vi "isi.vi"() -> ()   [LabVIEW 2019]
uses:
  <vilib>/DAQmx/write.llb/DAQmx Write (Digital Bool 1Line 1Point).vi
  <vilib>/DAQmx/read.llb/DAQmx Read (Analog 1D Wfm NChan NSamp).vi
  <vilib>/DAQmx/write.llb/DAQmx Write (Analog 1D DBL 1Chan NSamp).vi
  <vilib>/DAQmx/create/channels.llb/DAQmx Create Channel (DO-Digital Output).vi
  <vilib>/DAQmx/miscellaneous.llb/DAQmx Fill In Error Info.vi
  <vilib>/DAQmx/create/channels.llb/DAQmx Create Channel (AO-Voltage-Basic).vi
  <vilib>/DAQmx/configure/timing.llb/DAQmx Timing (Sample Clock).vi
  <vilib>/DAQmx/create/channels.llb/DAQmx Create Channel (AI-Voltage-Basic).vi
  <vilib>/DAQmx/configure/task.llb/DAQmx Configure Logging (TDMS).vi
  <vilib>/measure/NI_MABase.lvlib
panel:
  in  "确定按钮":bool
  in  "lines":tag="Dev2/port0/line0" caption="事件通道"
  in  "logging mode":i32(ring)=10231 caption="记录模式" items=["关"=10231, "记录"=15844, "记录并读取"=15842]
  out "波形图":waveform(dbl)[](graph)
  in  "samples per channel":i32=1000 caption="每通道采样"
  in  "physical channels":tag="Dev2/ai0:3" caption="输入通道"
  in  "file path":path caption="文件路径"
  in  "停止 2":bool
  in  "lines 2":tag="Dev2/port0/line1" caption="刺激事件通道"
  in  "胡须刺激":bool
  in  "frequency":dbl=10.0 caption="刺激频率" format="%0.2p"
  in  "amplitude":dbl=2.5 caption="刺激幅值" format="%0.2p"
  in  "physical channels 3":tag="Dev2/ao1" caption="胡须刺激通道"
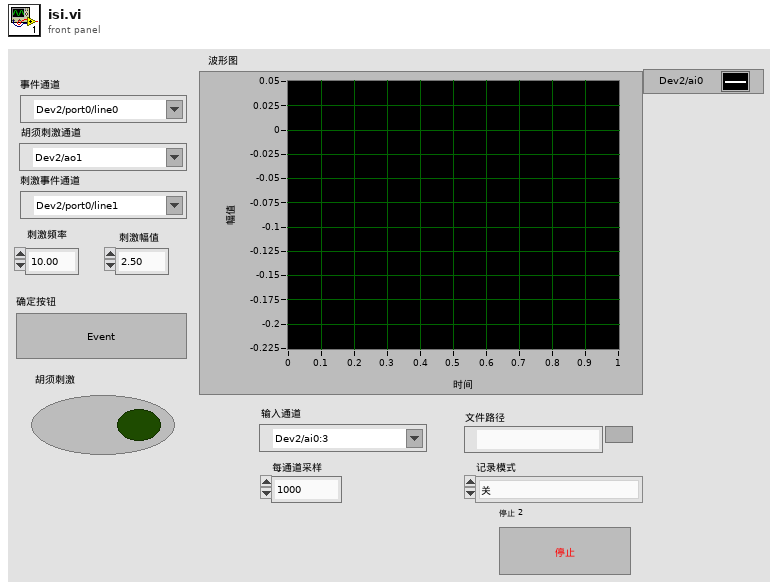
[diagram p1: front panel]
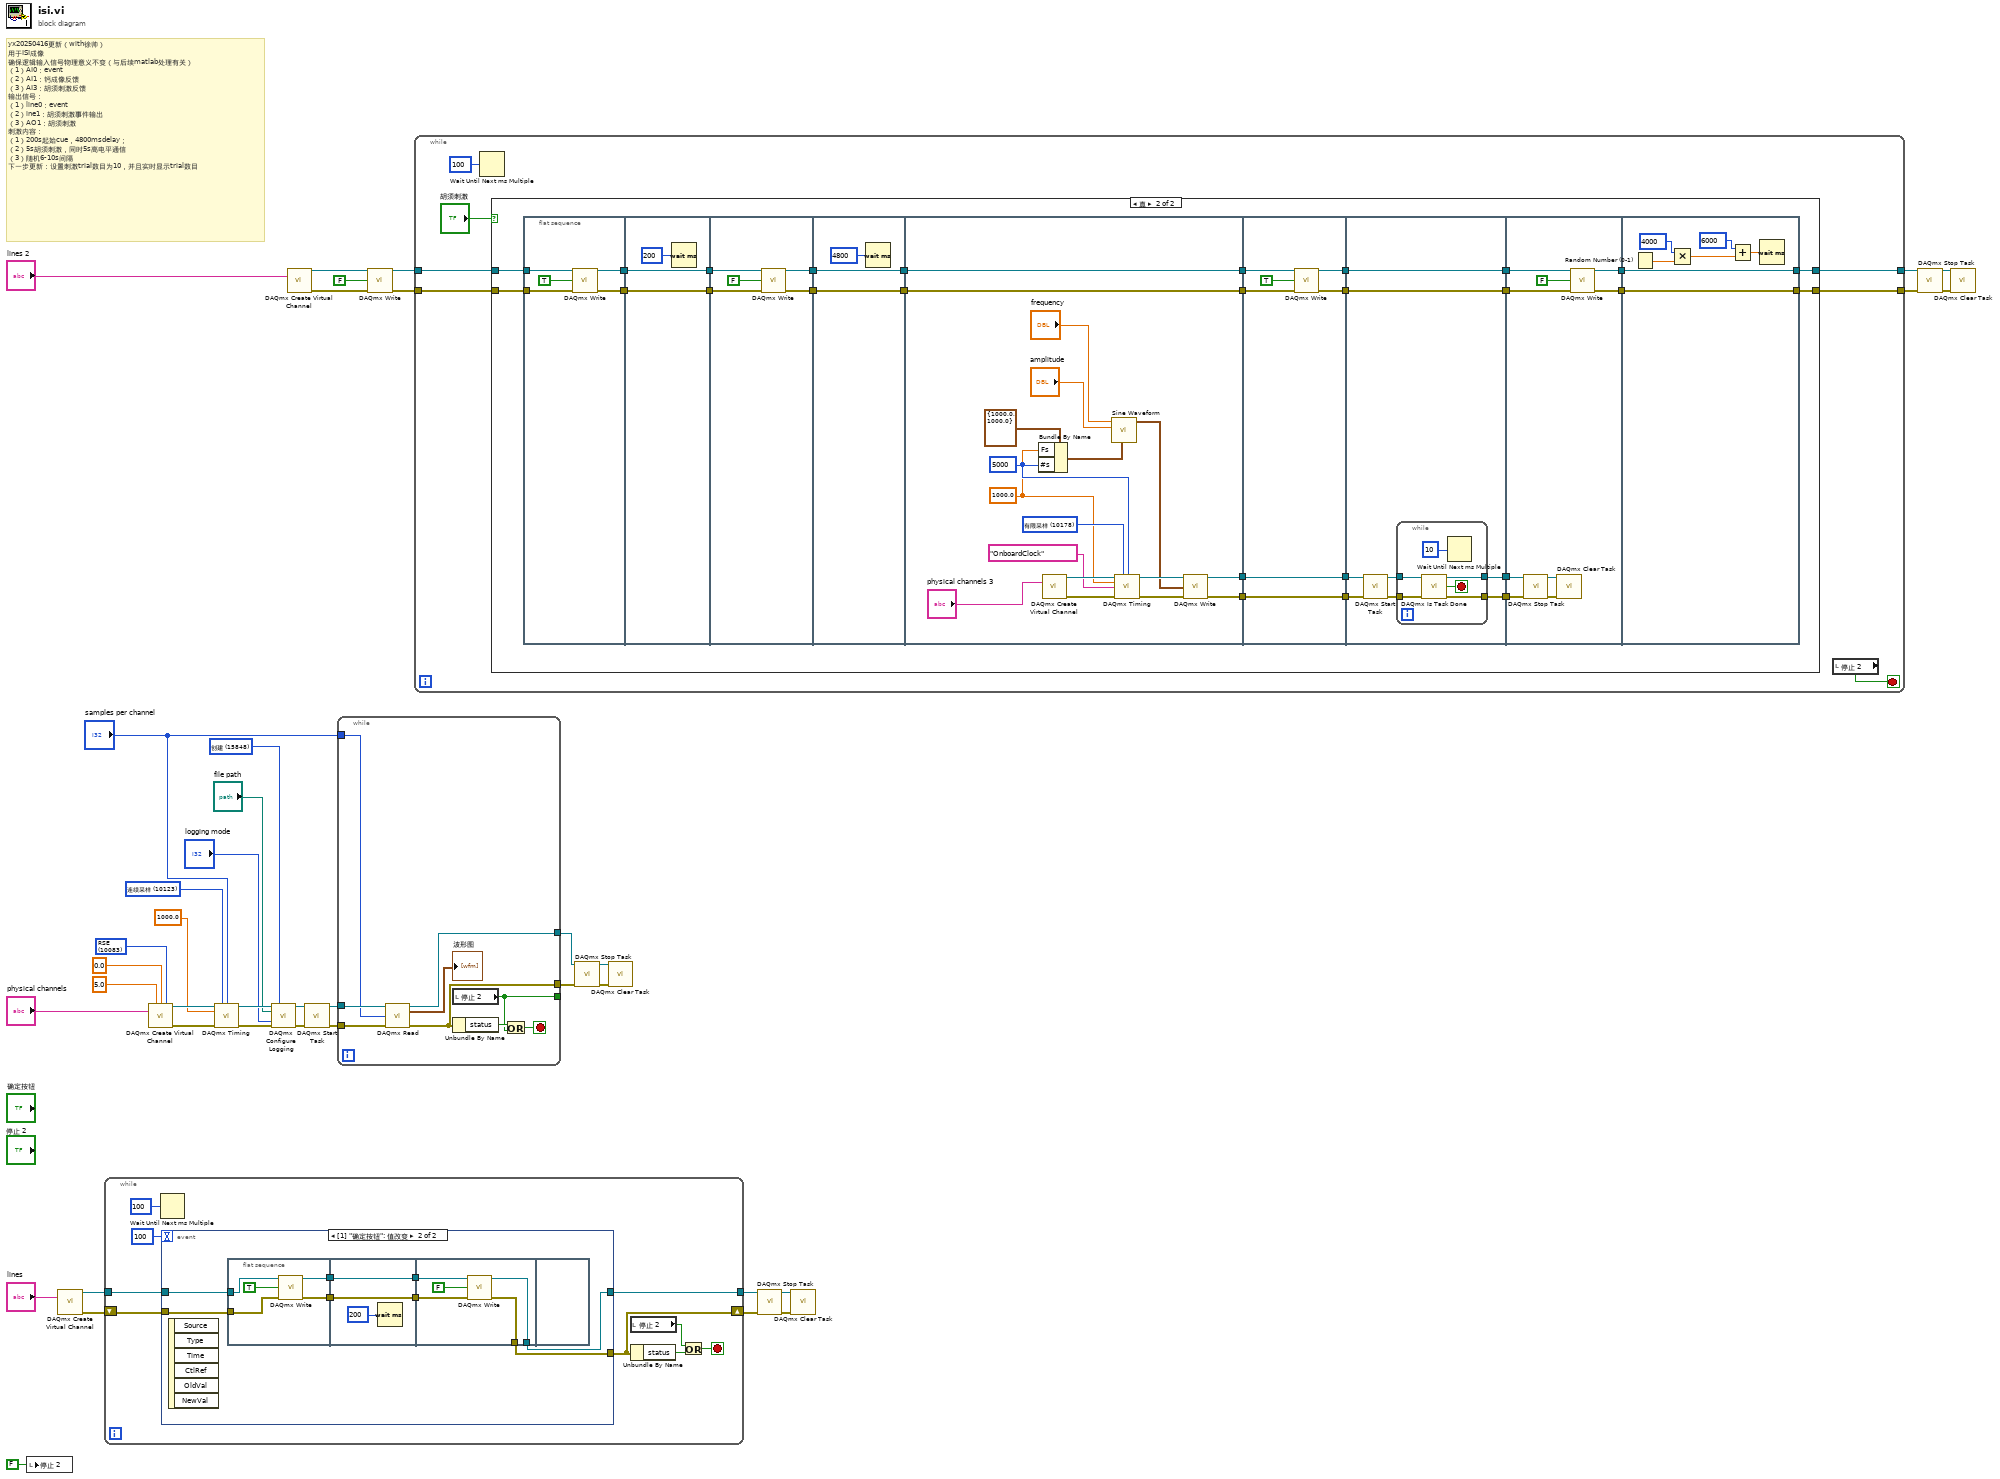
[diagram p0: block diagram]
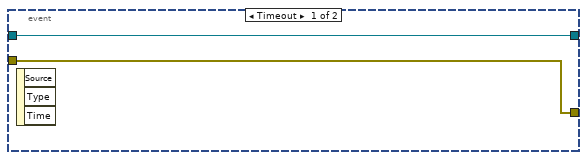
[diagram p2: hidden frame]
diagram:
  w3 = 10083 items=["默认"=-1, "RSE"=10083, "NRSE"=10078, "差分"=10106, "伪差分"=12529] ("input terminal configuration")
  w21 = 15848 items=["打开"=10437, "打开或创建"=15846, "创建或替换"=15847, "创建"=15848] ("operation")
  w25 = 10123 items=["有限采样"=10178, "连续采样"=10123, "硬件定时单点"=12522] ("sample mode")
  # "yx20250416更新（with徐帅）\n用于ISI成像\n确保逻辑输入信号物理意义不变（与后续matlab处理有关）\n（1）AI0：event\n（2）AI1：钙成像反馈\n（3）AI3：胡须刺激反馈\n输出信号：\n（1）line0：event\n（2）ine1：胡须刺激事件输出\n（3）AO1：胡须刺激\n刺激内容：\n（1）200s起始cue，4800msdelay；\n（2）5s胡须刺激，同时5s高电平通信\n（3）随机6-10s间隔\n下一步更新：设置刺激trial数目为10，并且实时显示trial数目"
  n1 = local write "停止 2"(FALSE) -> ()
  n2 = call-poly <vilib>:"DAQmx Create Virtual Channel.vi"("lines"="lines") -> ("task out"=w7:refnum<k21>, "error out"=w6:errorcluster)  [unwired: 13 in]
  n3 = while {
    shift-right: [w45] -> w4
    shift-left: w6 -> [w48]
    tunnel: w7 -> [w49]
    tunnel: [w47] -> w5
    stop <- w42 stop-if-true
    n4 = Wait Until Next ms Multiple(millisecond multiple=u32 100) -> ()  [unwired: 1 out]
    n5 = event shown="[1] \"确定按钮\": 值改变" {
      selector: _ -> [_ _]
      dyn-events: _ -> [_ _]
      timeout: 100 -> [_ _]
      tunnel: w49 -> [w51 w59]
      tunnel: w48 -> [w50 w56]
      tunnel: [w51 w53] -> w47
      tunnel: [w50 w52] -> w45
      event Timeout {
        n6 = event-data() -> ()  [unwired: 1 in, 3 out]
      }
      event "确定按钮": Value Change {
        n7 = event-data() -> ()  [unwired: 1 in, 6 out]
        n8 = flat-sequence {
          tunnel: w59 -> [w63]
          tunnel: [w62] -> w57
          tunnel: w56 -> [w61]
          tunnel: [w60] -> w54
          tunnel: [w66] -> w58
          tunnel: w57 -> [w66]
          tunnel: [w65] -> w55
          tunnel: w54 -> [w65]
          tunnel: w58 -> [w71]
          tunnel: w55 -> [w70]
          tunnel: [w69] -> w53
          tunnel: [w68] -> w52
          frame #0 {
            n9 = call-poly <vilib>:"DAQmx Write.vi"("task/channels in"=w63, "data"=TRUE, "error in"=w61) -> ("task out"=w62:refnum<k21>, "error out"=w60:errorcluster)  [unwired: 10 in, 1 out]
          }
          frame #1 {
            n10 = Wait (ms)(milliseconds to wait=u32 200 ("等待时间（毫秒）")) -> ()  [unwired: 1 out]
          }
          frame #2 {
            n11 = call-poly <vilib>:"DAQmx Write.vi"("task/channels in"=w71, "data"=FALSE, "error in"=w70) -> ("task out"=w69:refnum<k21>, "error out"=w68:errorcluster)  [unwired: 10 in, 1 out]
          }
          frame #3 {
          }
        }
      }
    }
    n12 = local read "停止 2"() -> (w43:bool)
    n13 = Unbundle By Name(w45) -> ("status"=w44:bool)
    n14 = Or(x=w43, y=w44) -> (x .or. y?=w42:bool)
  }
  n15 = call-poly <vilib>:"DAQmx Create Virtual Channel.vi"("maximum value"=5.0, "minimum value"=0.0, "input terminal configuration"=w3, "physical channels"="physical channels") -> ("task out"=w27:refnum<k21>, "error out"=w26:errorcluster)  [unwired: 10 in]
  n16 = call-poly <vilib>:"DAQmx Timing.vi"("task/channels in"=w27, "sample mode"=w25, "samples per channel"="samples per channel", "rate"=1000.0, "error in"=w26) -> ("task out"=w24:refnum<k21>, "error out"=w23:errorcluster)  [unwired: 9 in]
  n17 = call-poly <vilib>:"DAQmx Configure Logging.vi"("task/channels in"=w24, "operation"=w21, "file path"="file path", "logging mode"="logging mode", "error in"=w23) -> ("task out"=w20:refnum<k21>, "error out"=w19:errorcluster)  [unwired: 9 in]
  n18 = call-poly <vilib>:"DAQmx Create Virtual Channel.vi"("lines"="lines 2") -> ("task out"=w39:refnum<k21>, "error out"=w38:errorcluster)  [unwired: 13 in]
  n19 = call <vilib>:"DAQmx Start Task.vi"("task/channels in"=w20, "error in"=w19) -> ("task out"=w18:refnum<k21>, "error out"=w17:errorcluster)  [unwired: 12 in]
  n20 = while {
    tunnel: w18 -> [w79]
    tunnel: w17 -> [w78]
    tunnel: "samples per channel" -> [w77]
    tunnel: [w75] -> w15
    tunnel: [w74] -> w13
    tunnel: [w73] -> _
    stop <- w76 stop-if-true
    n21 = call-poly <vilib>:"DAQmx Read.vi"("task/channels in"=w79, "number of samples per channel"=w77, "error in"=w78) -> ("task out"=w75:refnum<k21>, "data"=→"波形图":waveform(dbl)[], "error out"=w74:errorcluster)  [unwired: 10 in]
    n22 = local read "停止 2"() -> (w73:bool)
    n23 = Unbundle By Name(w74) -> ("status"=w81:bool)
    n24 = Or(x=w81, y=w73) -> (x .or. y?=w76:bool)
  }
  n25 = call-poly <vilib>:"DAQmx Write.vi"("task/channels in"=w39, "data"=FALSE, "error in"=w38) -> ("task out"=w37:refnum<k21>, "error out"=w36:errorcluster)  [unwired: 10 in, 1 out]
  n26 = while {
    tunnel: w37 -> [w86]
    tunnel: w36 -> [w85]
    tunnel: [w84] -> w32
    tunnel: [w83] -> w31
    stop <- w87 stop-if-true
    n27 = Wait Until Next ms Multiple(millisecond multiple=u32 100) -> ()  [unwired: 1 out]
    n28 = case shown="真" "胡须刺激" {
      tunnel: w86 -> [w90 w116]
      tunnel: w85 -> [w89 w115]
      tunnel: [w90 w114] -> w84
      tunnel: [w89 w113] -> w83
      frame False {
      }
      frame True {
        n29 = flat-sequence {
          tunnel: w116 -> [w121]
          tunnel: w115 -> [w120]
          tunnel: [w119] -> w98
          tunnel: [w118] -> w96
          tunnel: w98 -> [w124]
          tunnel: [w124] -> w97
          tunnel: w96 -> [w123]
          tunnel: [w123] -> w95
          tunnel: w97 -> [w129]
          tunnel: w95 -> [w128]
          tunnel: [w126] -> w94
          tunnel: [w125] -> w92
          tunnel: w94 -> [w132]
          tunnel: [w132] -> w93
          tunnel: w92 -> [w131]
          tunnel: [w131] -> w91
          tunnel: [w139] -> w112
          tunnel: [w138] -> w110
          tunnel: [w137] -> w108
          tunnel: w93 -> [w137]
          tunnel: [w136] -> w107
          tunnel: w91 -> [w136]
          tunnel: w112 -> [w157]
          tunnel: [w157] -> w111
          tunnel: w110 -> [w156]
          tunnel: [w156] -> w109
          tunnel: w108 -> [w154]
          tunnel: w107 -> [w152]
          tunnel: [w153] -> w106
          tunnel: [w151] -> w105
          tunnel: w111 -> [w163]
          tunnel: w109 -> [w162]
          tunnel: [w161] -> w104
          tunnel: [w160] -> w103
          tunnel: [w159] -> w102
          tunnel: [w158] -> w101
          tunnel: w106 -> [w159]
          tunnel: w105 -> [w158]
          tunnel: w104 -> [w173]
          tunnel: w103 -> [w172]
          tunnel: w102 -> [w179]
          tunnel: w101 -> [w177]
          tunnel: [w178] -> w100
          tunnel: [w176] -> w99
          tunnel: [w182] -> w114
          tunnel: [w181] -> w113
          tunnel: w100 -> [w182]
          tunnel: w99 -> [w181]
          frame #0 {
            n30 = call-poly <vilib>:"DAQmx Write.vi"("task/channels in"=w121, "data"=TRUE, "error in"=w120) -> ("task out"=w119:refnum<k21>, "error out"=w118:errorcluster)  [unwired: 10 in, 1 out]
          }
          frame #1 {
            n31 = Wait (ms)(milliseconds to wait=u32 200 ("等待时间（毫秒）")) -> ()  [unwired: 1 out]
          }
          frame #2 {
            n32 = call-poly <vilib>:"DAQmx Write.vi"("task/channels in"=w129, "data"=FALSE, "error in"=w128) -> ("task out"=w126:refnum<k21>, "error out"=w125:errorcluster)  [unwired: 10 in, 1 out]
          }
          frame #3 {
            n33 = Wait (ms)(milliseconds to wait=u32 4800 ("等待时间（毫秒）")) -> ()  [unwired: 1 out]
          }
          frame #4 {
            w148 = 10178 items=["有限采样"=10178, "连续采样"=10123, "硬件定时单点"=12522] ("sample mode")
            w144 = 1000.0 ("rate")
            w145 = 5000 ("samples per channel")
            n34 = Bundle By Name(cluster=cluster{"Fs":dbl, "#s":dbl} {"Fs"=1000.0, "#s"=1000.0} ("sampling info"), "Fs"=w144, "#s"=w145) -> (w143:cluster{"Fs":dbl, "#s":dbl})
            n35 = call-poly <vilib>:"DAQmx Create Virtual Channel.vi"("physical channels"="physical channels 3") -> ("task out"=w149:refnum<k21>, "error out"=w150:errorcluster)  [unwired: 13 in]
            n36 = call <vilib>:"Sine Waveform.vi"("sampling info"=w143, "amplitude"="amplitude", "frequency"="frequency") -> ("signal out"=w140:waveform(dbl))  [unwired: 7 in, 1 out]
            n37 = call-poly <vilib>:"DAQmx Timing.vi"("task/channels in"=w149, "sample mode"=w148, "samples per channel"=w145, "rate"=w144, "source"=tag "OnboardClock", "error in"=w150) -> ("task out"=w142:refnum<k21>, "error out"=w141:errorcluster)  [unwired: 8 in]
            n38 = call-poly <vilib>:"DAQmx Write.vi"("task/channels in"=w142, "data"=w140, "error in"=w141) -> ("task out"=w139:refnum<k21>, "error out"=w138:errorcluster)  [unwired: 10 in, 1 out]
          }
          frame #5 {
            n39 = call-poly <vilib>:"DAQmx Write.vi"("task/channels in"=w154, "data"=TRUE, "error in"=w152) -> ("task out"=w153:refnum<k21>, "error out"=w151:errorcluster)  [unwired: 10 in, 1 out]
          }
          frame #6 {
            n40 = call <vilib>:"DAQmx Start Task.vi"("task/channels in"=w163, "error in"=w162) -> ("task out"=w164:refnum<k21>, "error out"=w165:errorcluster)  [unwired: 12 in]
            n41 = while {
              tunnel: w164 -> [w170]
              tunnel: [w169] -> w161
              tunnel: w165 -> [w168]
              tunnel: [w167] -> w160
              stop <- w171 stop-if-true
              n42 = call <vilib>:"DAQmx Is Task Done.vi"("task/channels in"=w170, "error in"=w168) -> ("task out"=w169:refnum<k21>, "task done?"=w171:bool, "error out"=w167:errorcluster)  [unwired: 11 in]
              n43 = Wait Until Next ms Multiple(millisecond multiple=u32 10) -> ()  [unwired: 1 out]
            }
          }
          frame #7 {
            n44 = call <vilib>:"DAQmx Stop Task.vi"("task/channels in"=w173, "error in"=w172) -> ("task out"=w174:refnum<k21>, "error out"=w175:errorcluster)  [unwired: 12 in]
            n45 = call <vilib>:"DAQmx Clear Task.vi"("task in"=w174, "error in"=w175) -> ()  [unwired: 13 in, 1 out]
            n46 = call-poly <vilib>:"DAQmx Write.vi"("task/channels in"=w179, "data"=FALSE, "error in"=w177) -> ("task out"=w178:refnum<k21>, "error out"=w176:errorcluster)  [unwired: 10 in, 1 out]
          }
          frame #8 {
            n47 = Random Number (0-1)() -> (number: 0 to 1=w187:dbl)
            n48 = Multiply(x=u32 4000 ("等待时间（毫秒）"), y=w187) -> (x*y=w185:dbl)
            n49 = Add(x=u32 6000 ("等待时间（毫秒）"), y=w185) -> (x+y=w183:dbl)
            n50 = Wait (ms)(milliseconds to wait=w183) -> ()  [unwired: 1 out]
          }
        }
      }
    }
    n51 = local read "停止 2"() -> (w87:bool)
  }
  n52 = call <vilib>:"DAQmx Stop Task.vi"("task/channels in"=w15, "error in"=w13) -> ("task out"=w14:refnum<k21>, "error out"=w12:errorcluster)  [unwired: 12 in]
  n53 = call <vilib>:"DAQmx Clear Task.vi"("task in"=w14, "error in"=w12) -> ()  [unwired: 13 in, 1 out]
  n54 = call <vilib>:"DAQmx Stop Task.vi"("task/channels in"=w5, "error in"=w4) -> ("task out"=w2:refnum<k21>, "error out"=w1:errorcluster)  [unwired: 12 in]
  n55 = call <vilib>:"DAQmx Clear Task.vi"("task in"=w2, "error in"=w1) -> ()  [unwired: 13 in, 1 out]
  n56 = call <vilib>:"DAQmx Stop Task.vi"("task/channels in"=w32, "error in"=w31) -> ("task out"=w34:refnum<k21>, "error out"=w33:errorcluster)  [unwired: 12 in]
  n57 = call <vilib>:"DAQmx Clear Task.vi"("task in"=w34, "error in"=w33) -> ()  [unwired: 13 in, 1 out]
